vi "Single_Core_Noise_Img_Gen.vi"(8 "error IN":errorcluster, 9 "[IN] Width":i32, 10 "[IN] Height":i32) -> (0 "error OUT":errorcluster, 2 "[OUT] U16 Pixel Img":u16[][](array[numeric]))   [LabVIEW 2020]
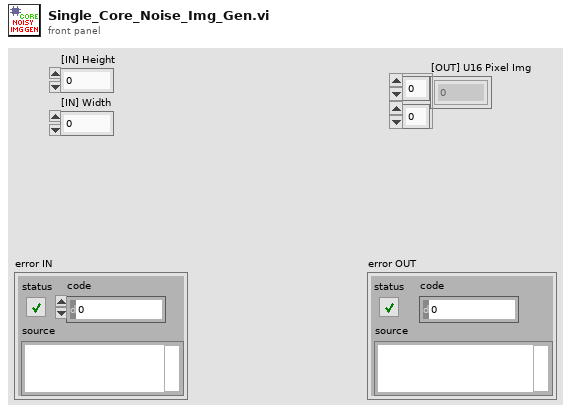
[diagram p1: front panel]
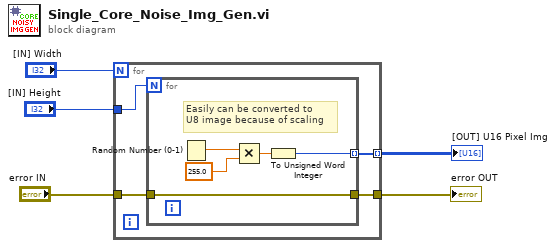
[diagram p0: block diagram]
diagram:
  n1 = for {
    N: "[IN] Width" -> [_]
    tunnel: "[IN] Height" -> [w9]
    tunnel: [w8] -> w3 mode=indexing
    tunnel: "error IN" -> [w7]
    tunnel: [w6] -> w4
    n2 = for {
      N: w9 -> [_]
      tunnel: [w11] -> w8 mode=indexing
      tunnel: w7 -> [w10]
      tunnel: [w10] -> w6
      # "Easily can be converted to\nU8 image because of scaling"
      n3 = Random Number (0-1)() -> (number: 0 to 1=w14:dbl)
      n4 = Multiply(x=w14, y=255.0) -> (x*y=w12:dbl)
      n5 = To Unsigned Word Integer(number=w12) -> (unsigned 16bit integer=w11:u16)
    }
  }
  "error OUT" <- w4
  "[OUT] U16 Pixel Img" <- w3
